vi "MAIN_merFISH_laser_scan.vi"(3 "queue DAQ":refnum<queue>, 5 "queue CAMERA":refnum<queue>, 7 "queue piezo":refnum<queue>, 8 "error in":errorcluster, 9 "Display?":bool=TRUE, 10 "Exp time (s)":sgl=0.05 format="%#_3g", 11 "DATA cluster":T2) -> (0 "error out":errorcluster, 1 "Next task":T1)   [LabVIEW 2015]
uses:
  CONTROLS/Q_MCL_piezo_element.ctl
  CONTROLS/Q_DAQ_element.ctl
  CONTROLS/Q_main_element.ctl
  CONTROLS/Q_camera_element.ctl
  GLOBAL/Global_MCL_piezo.vi
  GLOBAL/Global_ABORT.vi
  GLOBAL/Global_MAIN.vi
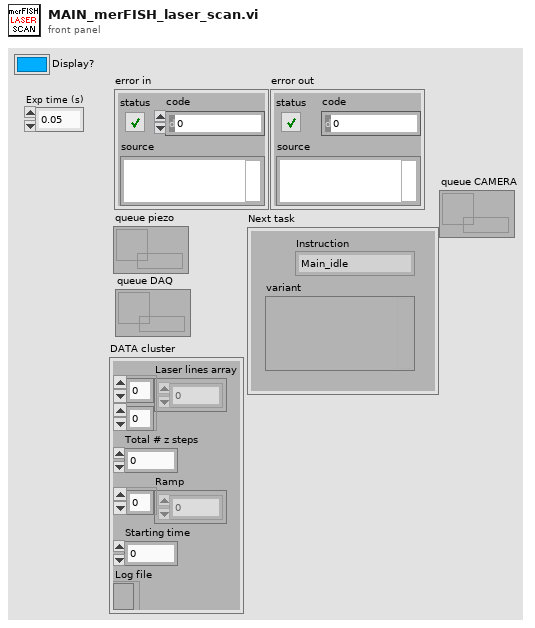
[diagram p1: front panel]
types:
  T1 = typedef "Q_main_element.ctl" = cluster{"variant":variant, "Instruction":enum16{"Main_idle", "Main_initialize", "Main_initialize_TDMS", "Main_initialize_Queue", "Main_error", "Main_DAQ_initialization_results", "Main_ASI_initialization_results", "Main_Piezo_initialization_results", "Main_Valve_initialization_results", "Main_Pump_initialization_results", "Main_CAMERA_initialization_results", "Main_FPGA_initialization_results", "Main_DAQ_error", "Main_ASI_error", "Main_Piezo_error", "Main_CAMERA_error", "Main_Valve_error", "Main_Pump_error", "Main_FPGA_error", "Main_start_acquiring", "Main_not_acquiring", "Main_acquiring", "Main_stop_acquiring", "Main_change_exposure", "Main_change_z_scan_parameters", "Main_define_ROI", "Main_define_mosaic", "Main_read_kinetic_time", "Main_cooler", "Main_read_temperature", "Main_save_XY", "Main_load_XY", "Main_discard_XY", "Main_move_to_XY", "Main_measure_QPD", "Main_autofocus_calibration", "Main_autofocus_initialization", "Main_autofocus_stop", "Main_save_PID", "Main_change_H_valve_position", "Main_two_way_valve", "Main_save_movie", "Main_init_single_scan", "Main_single_scan", "Main_stop_single_scan", "Main_merFISH_illumination_parameters", "Main_merFISH_buffer_probe_list", "Main_merFISH_injections_procedure", "Main_merFISH_save_setpoint", "Main_merFISH_DAPI_parameters", "Main_merFISH_Brightfield_parameters", "Main_merFISH_save_embryo_ROI", "Main_merFISH_init", "Main_merFISH_resume", "Main_merFISH_start_autofocus", "Main_merFISH_open_close_valve_merFISH", "Main_merFISH_open_close_valve_photobleaching", "Main_merFISH_hybridization", "Main_merFISH_move_to_ROI", "Main_merFISH_wait_stabilization", "Main_merFISH_scan_laser", "Main_merFISH_scan_brightfield", "Main_merFISH_photobleaching_injection", "Main_merFISH_photobleaching", "Main_merFISH_save", "Main_merFISH_send_email", "Main_merFISH_close", "Main_STOP"}}
  T2 = cluster{"Laser lines array":dbl[][], "Total # z steps":i32, "Ramp":dbl[], "Starting time":dbl, "Log file":refnum<file>}
  T3 = typedef "Q_MCL_piezo_element.ctl" = cluster{"variant":variant, "Instruction":enum16{"Piezo_idle", "Piezo_initialize", "Piezo_error", "Piezo_security_stop", "Piezo_read_z", "Piezo_move_z", "Piezo_keyboard_move", "Piezo_close_autofocus_calibration_ramp", "Piezo_change_init_state", "Piezo_init_autofocus", "Piezo_init_autofocus_merFISH_TL", "Piezo_autofocus", "Piezo_autofocus_merFISH_TL", "Piezo_stop_autofocus", "Piezo_stop_autofocus_merFISH_TL", "Piezo_autofocus_lost", "Piezo_resume_autofocus_merFISH_TL", "Piezo_check_z_position_merFISH_TL", "Piezo_init_ramp", "Piezo_move_z_ramp", "Piezo_close_ramp", "Piezo_close_merFISH", "Piezo_stop"}}
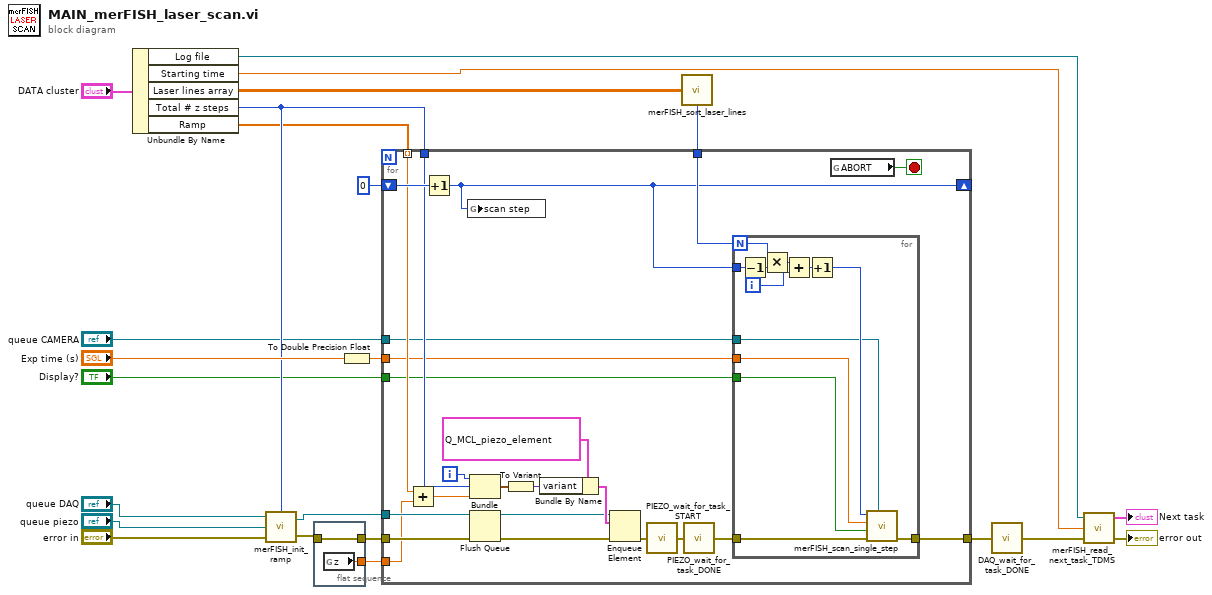
[diagram p0: block diagram]
diagram:
  n1 = Unbundle By Name("DATA cluster") -> ("Log file"=w2:refnum<file>, "Starting time"=w3:dbl, "Laser lines array"=w6:dbl[][], "Total # z steps"=w8:i32, "Ramp"=w7:dbl[])
  n2 = call "merFISH_init_ramp.vi"("Total # z steps"=w8, "error in"="error in", "Piezo queue"="queue piezo", "DAQ queue"="queue DAQ") -> ("error out"=w20:errorcluster, "Piezo queue out"=w21:refnum<queue>)
  n3 = flat-sequence {
    tunnel: [w25] -> w19
    tunnel: w20 -> [w24]
    tunnel: [w24] -> w17
    frame #0 {
      n4 = global read "Global_MCL_piezo.vi" "z"() -> (w25:dbl)
    }
  }
  n5 = To Double Precision Float(number="Exp time (s)") -> (double precision float=w23:dbl)
  n6 = call "merFISH_sort_laser_lines.vi"("Laser lines array"=w6) -> ("N laser lines merFISH"=w5:i32)  [unwired: 2 in, 2 out]
  n7 = for {
    tunnel: w7 -> [w32] mode=indexing
    tunnel: w8 -> [w40]
    shift-right: [w26] -> _
    shift-left: 0 -> [w42]
    tunnel: [w39] -> w18
    tunnel: w21 -> [w37]
    tunnel: w17 -> [w36]
    tunnel: w23 -> [w31]
    tunnel: w19 -> [w30]
    tunnel: w5 -> [w29]
    tunnel: "Display?" -> [w28]
    tunnel: "queue CAMERA" -> [w27]
    i -> [w43]
    stop <- w38 stop-if-true
    n8 = Add(x=w32, y=w30) -> (x+y=w33:dbl)
    n9 = Increment(x=w42) -> (x+1=w26:i32)
    n10 = global write "Global_MAIN.vi" "scan step"(w26) -> ()
    n11 = Bundle(w43, "Total # z steps"=w40, w33) -> (w49:cluster{i32, "Total # z steps":i32, dbl})  [unwired: 1 in]
    n12 = Flush Queue(queue=w37, error in (no error)=w36) -> (queue out=w35:refnum<queue>, error out=w34:errorcluster)  [unwired: 1 out]
    n13 = To Variant(anything=w49) -> (Variant=w45:variant)
    n14 = Bundle By Name(cluster=T3 {"variant"=variant, "Instruction"=enum."Piezo_move_z_ramp"} ("Q_MCL_Piezo"), "variant"=w45) -> (w46:T3)
    n15 = Enqueue Element(queue=w35, element=w46, error in (no error)=w34) -> (error out=w47:errorcluster)  [unwired: 1 in, 2 out]
    n16 = call "PIEZO_wait_for_task_START.vi"("error in"=w47) -> ("error out"=w48:errorcluster)
    n17 = call "PIEZO_wait_for_task_DONE.vi"("error in"=w48) -> ("error out"=w41:errorcluster)
    n18 = for {
      N: w29 -> [w56]
      tunnel: w41 -> [w61]
      tunnel: w26 -> [w57]
      tunnel: [w51] -> w39
      tunnel: w31 -> [w53]
      tunnel: w28 -> [w52]
      tunnel: w27 -> [w50]
      i -> [w55]
      n19 = Decrement(x=w57) -> (x-1=w60:i32)
      n20 = Multiply(x=w56, y=w60) -> (x*y=w58:i32)
      n21 = Add(x=w58, y=w55) -> (x+y=w59:i32)
      n22 = Increment(x=w59) -> (x+1=w54:i32)
      n23 = call "merFISH_scan_single_step.vi"("queue CAMERA"=w50, "error in"=w61, "Display?"=w52, "Pulse length Ton (s)"=w53, "image #"=w54) -> ("error out"=w51:errorcluster)  [unwired: 3 in]
    }
    n24 = global read "Global_ABORT.vi" "ABORT"() -> (w38:bool)
  }
  n25 = call "DAQ_wait_for_task_DONE.vi"("error in"=w18) -> ("error out"=w22:errorcluster)
  n26 = call "merFISH_read_next_task_TDMS.vi"("error in"=w22, "Starting time"=w3, "Log file"=w2) -> ("error out"=→"error out":errorcluster, "task"=→"Next task":T1)  [unwired: 1 in]
